vi "Autonomous Independent.vi"() -> ()   [LabVIEW 2012]
doc: "This VI is called when autonomous begins, and will automatically be terminated when autonomous ends. You can carry out timed or sensor driven robot movement independently without needing to return to the caller."
uses:
  <vilib>/Rock Robotics/WPI/Solenoid/WPI_SolenoidValue.ctl
  Robot Global Data.vi
  <vilib>/Rock Robotics/WPI/Solenoid/WPI_SolenoidSetEnum.vi
  <vilib>/Rock Robotics/WPI/Joystick/WPI_JoystickGetSetRefNum.vi
panel:
  in  "Shooter power 2":dbl=1.0
  in  "Shooter power":dbl=1.0
  in  "stop":bool
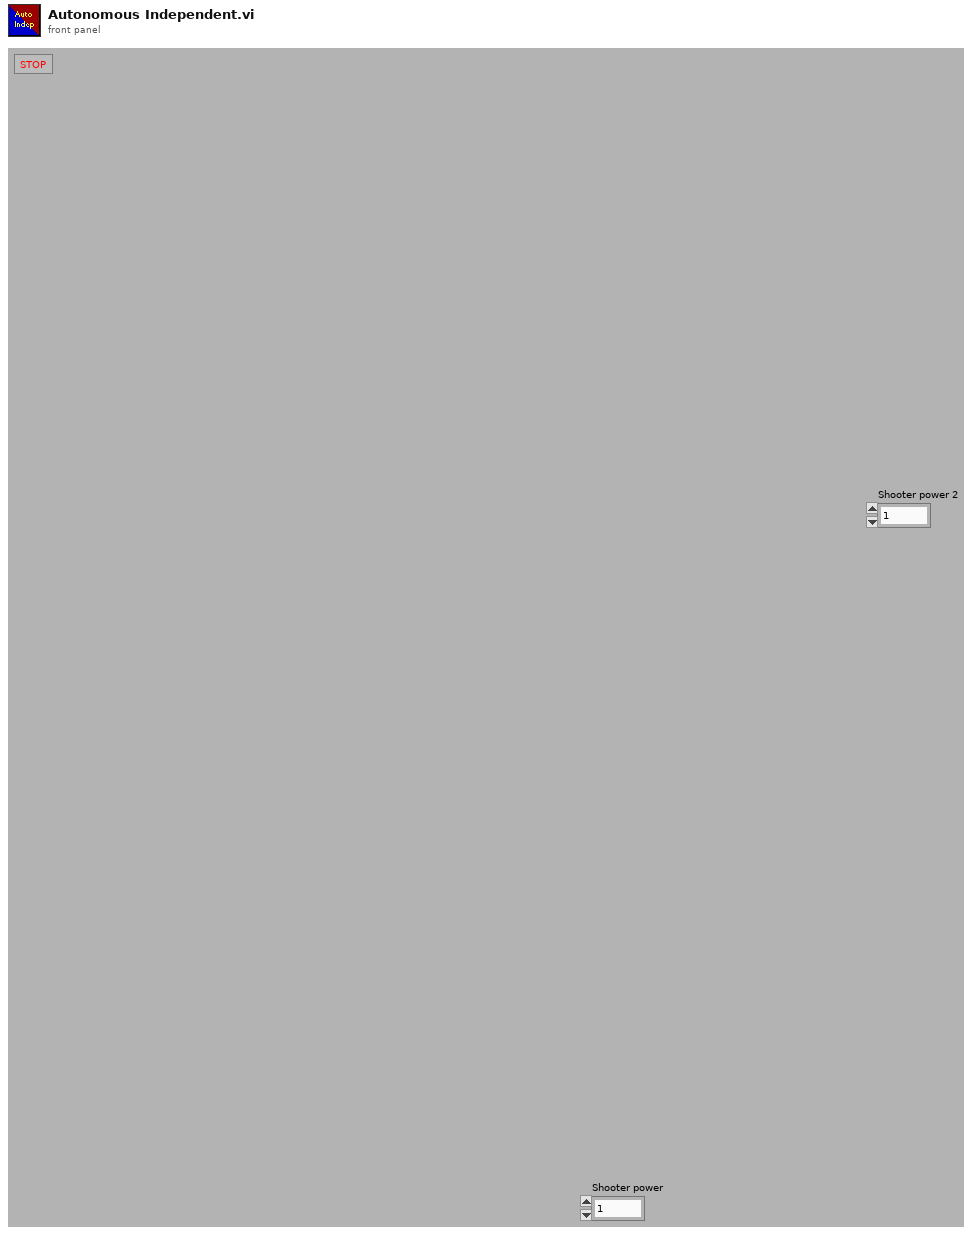
[diagram p1: front panel]
types:
  T1 = typedef "WPI_JoystickDevRef.ctl" = cluster{"Device":T2}
  T2 = typedef "WPI_JoystickDeviceEnum.ctl" = enum16{"USB 1", "USB 2", "USB 3", "USB 4", "Kinect 1", "Kinect 2"}
  T3 = cluster{"axis 1 (x)":dbl, "axis 2 (y)":dbl, "axis 3 (throttle)":dbl, "axis 4":dbl, "axis 5":dbl, "axis 6":dbl}
  T4 = typedef "WPI_SolenoidValue.ctl" = enum16{"Off", "On", "Forward", "Reverse"}
  T5 = typedef "WPI_MotorControlDeviceRef.ctl" = cluster{"DeviceStatus":errorcluster, "Type":enum16{"PWM", "CAN"}, "PWM":cluster{"Digital Module":T6, "PWM Channel":T7, "DeadBand":T8}, "CAN":cluster{"Device Number":u8, "Control Mode":T9, "Semaphore":T10, "Max Vout":dbl}, "Invert":bool, "TransformRef":T11, "InvTransformRef":T11}
  T6 = typedef "FPGA_TypedefDigitalModule.ctl" = enum16{"Digital Module 1", "Digital Module 2"}
  T7 = typedef "FPGA_DIOPWMChannel.ctl" = enum8{"PWM 1", "PWM 2", "PWM 3", "PWM 4", "PWM 5", "PWM 6", "PWM 7", "PWM 8", "PWM 9", "PWM 10", "Invalid"}
  T8 = typedef "WPI_PWMDeadband.ctl" = cluster{"Name":string, "maxPositivePwm":i32, "minPositivePwm":i32, "centerPwm":i32, "maxNegativePwm":i32, "minNegativePwm":i32, "angularRange":u16}
  T9 = typedef "WPI_CANJaguar_ControlMode.ctl" = enum8{"Percent VBus", "Current", "Speed", "Position", "Voltage"}
  T10 = typedef "Semaphore RefNum" = refnum<k1>
  T11 = typedef "WPI_PWMTransform_ConPane.ctl" = refnum<vi>
  T12 = typedef "WPI_SolenoidDevRef.ctl" = cluster{"DevStatus":errorcluster, "Solenoid Module":T13, "Forward Solenoid Channel":T14, "Reverse Solenoid Channel":T14}
  T13 = typedef "FPGA_TypedefSolenoidModule.ctl" = enum16{"Solenoid Module 1", "Solenoid Module 2"}
  T14 = typedef "WPI_SolenoidChannel.ctl" = enum8{"Solenoid 1", "Solenoid 2", "Solenoid 3", "Solenoid 4", "Solenoid 5", "Solenoid 6", "Solenoid 7", "Solenoid 8", "Invalid"}
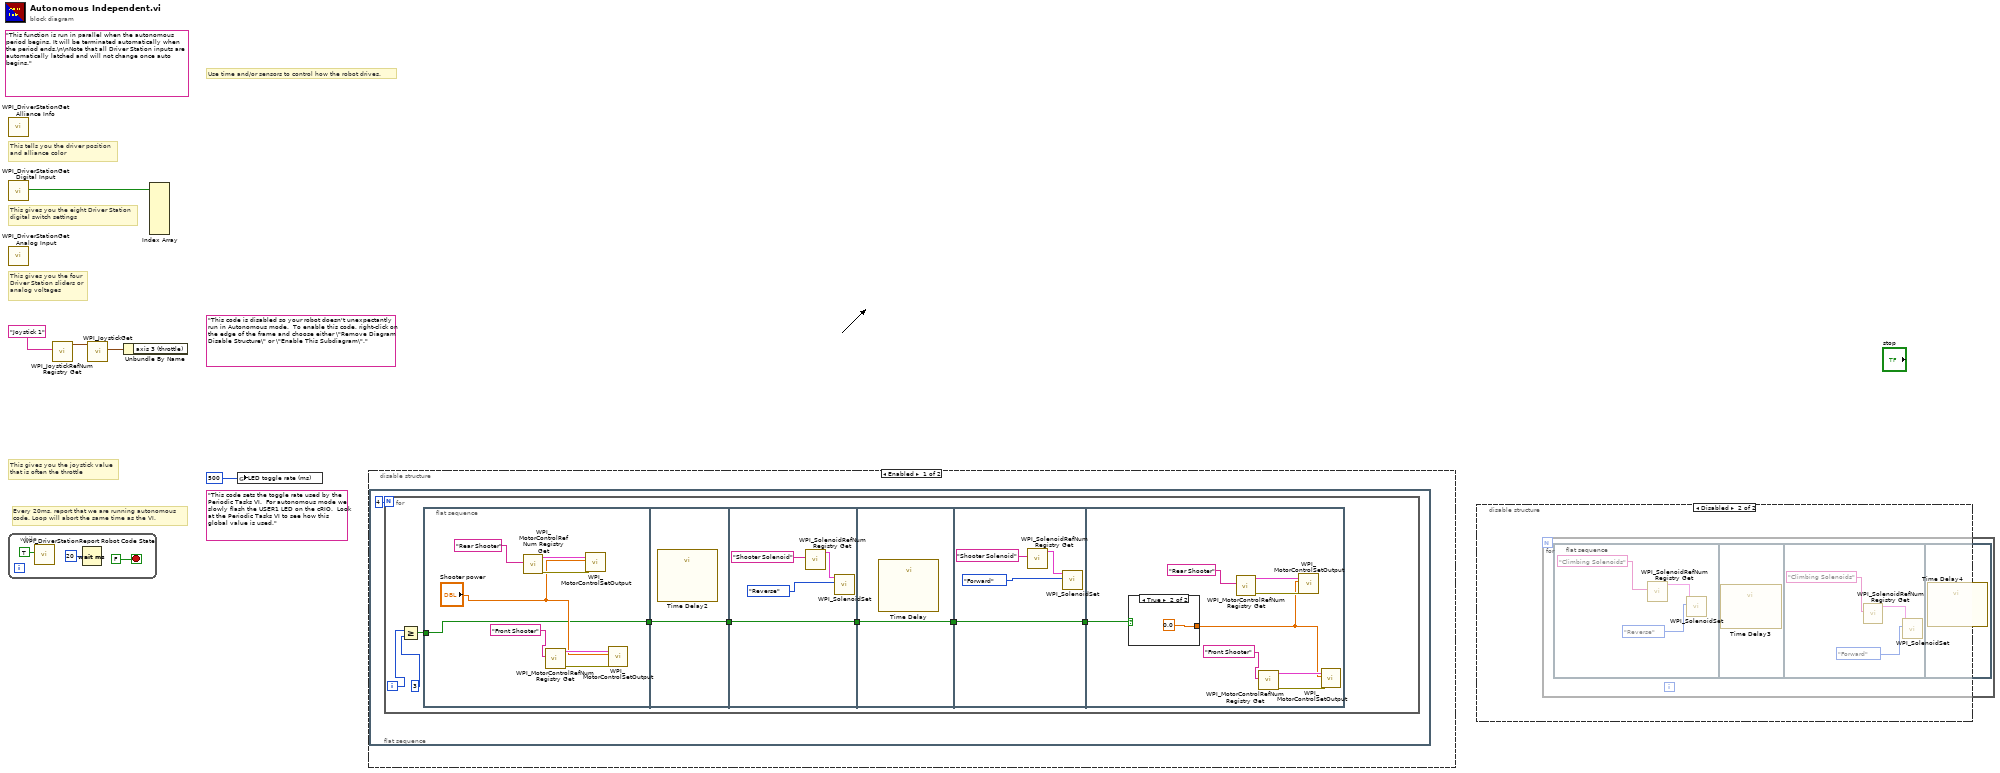
[diagram p0: block diagram]
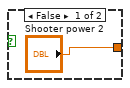
[diagram p3: hidden frame]
diagram:
  (unwired) "This code sets the toggle rate used by the Periodic Tasks VI.  For autonomous mode we slowly flash the USER1 LED on the cRIO.  Look at the Periodic Tasks VI to see how this global value is used."
  (unwired) "This code is disabled so your robot doesn't unexpectantly run in Autonomous mode.  To enable this code, right-click on the edge of the frame and choose either \"Remove Diagram Disable Structure\" or \"Enable This Subdiagram\"."
  (unwired) "This function is run in parallel when the autonomous period begins. It will be terminated automatically when the period ends.\n\nNote that all Driver Station inputs are automatically latched and will not change once auto begins."
  # "Every 20ms, report that we are running autonomous\ncode. Loop will abort the same time as the VI."
  # "This gives you the joystick value\nthat is often the throttle"
  # "Use time and/or sensors to control how the robot drives."
  # "This tells you the driver position\nand alliance color"
  # "This gives you the eight Driver Station\ndigital switch settings"
  # "This gives you the four\nDriver Station sliders or\nanalog voltages"
  n1 = while {
    stop <- FALSE stop-if-true
    n2 = call <vilib>:"WPI_DriverStationReport Robot Code State.vi"("Autonomous"=TRUE) -> ()  [unwired: 10 in, 1 out]
    n3 = Wait (ms)(milliseconds to wait=u32 20) -> ()  [unwired: 1 out]
  }
  n4 = call <vilib>:"WPI_DriverStationGet Alliance Info.vi"() -> ()  [unwired: 12 out]
  n5 = call <vilib>:"WPI_DriverStationGet Digital Input.vi"() -> ("Driver Station Digital Input (1-8)"=w5:bool[])  [unwired: 11 out]
  n6 = call <vilib>:"WPI_DriverStationGet Analog Input.vi"() -> ()  [unwired: 12 out]
  n7 = call <vilib>:"WPI_JoystickRefNum Registry Get.vi"("refnum name"="Joystick 1") -> ("JoystickDevRef"=w2:T1)  [unwired: 1 in, 9 out]
  n8 = call <vilib>:"WPI_JoystickGet.vi"("JoystickDevRef"=w2) -> ("Axes"=w3:T3)  [unwired: 1 in, 5 out]
  n9 = Unbundle By Name(w3) -> ()  [unwired: 1 out]
  n10 = Index Array(array=w5) -> ()  [unwired: 8 in, 8 out]
  n11 = global write "Robot Global Data.vi" "LED toggle rate (ms)"(u32 500 ("LED ms toggle rate")) -> ()
  n12 = disable-structure shown="Enabled" {
    frame Enabled {
      n13 = flat-sequence {
        frame #0 {
          n14 = for {
            N: 4 -> [_]
            i -> [w17]
            n15 = Greater Or Equal?(x=w17, y=3) -> (x >= y?=w10:bool)
            n16 = flat-sequence {
              tunnel: [w19] -> w16
              tunnel: w10 -> [w19]
              tunnel: w16 -> [w26]
              tunnel: [w26] -> w15
              tunnel: w15 -> [w27]
              tunnel: [w27] -> w14
              tunnel: w14 -> [w31]
              tunnel: [w31] -> w13
              tunnel: w13 -> [w32]
              tunnel: [w32] -> w12
              tunnel: w12 -> [w37]
              frame #0 {
                n17 = call <vilib>:"WPI_MotorControlRefNum Registry Get.vi"("refnum name"="Rear Shooter") -> ("error out"=w24:errorcluster, "MotorControlDevRef"=w25:T5)  [unwired: 9 in]
                n18 = call <vilib>:"WPI_MotorControlRefNum Registry Get.vi"("refnum name"="Front Shooter") -> ("error out"=w18:errorcluster, "MotorControlDevRef"=w23:T5)  [unwired: 9 in]
                n19 = call <vilib>:"WPI_MotorControlSetOutput.vi"("error in (no error)"=w24, "Output"="Shooter power", "MotorControlDevRef"=w25) -> ()  [unwired: 6 in, 3 out]
                n20 = call <vilib>:"WPI_MotorControlSetOutput.vi"("error in (no error)"=w18, "Output"="Shooter power", "MotorControlDevRef"=w23) -> ()  [unwired: 6 in, 3 out]
              }
              frame #1 {
                n21 = call "Time Delay2"() -> ()  [unwired: 11 in, 1 out]
              }
              frame #2 {
                n22 = call <vilib>:"WPI_SolenoidRefNum Registry Get.vi"("refnum name"="Shooter Solenoid") -> ("SolenoidDevRef"=w28:T12)  [unwired: 9 in, 1 out]
                n23 = call-poly <vilib>:"WPI_SolenoidSet.vi"("Value"=WPI_SolenoidValue."Reverse", "SolenoidDevRef"=w28) -> ()  [unwired: 8 in, 2 out]
              }
              frame #3 {
                n24 = call "Time Delay"() -> ()  [unwired: 11 in, 1 out]
              }
              frame #4 {
                n25 = call <vilib>:"WPI_SolenoidRefNum Registry Get.vi"("refnum name"="Shooter Solenoid") -> ("SolenoidDevRef"=w35:T12)  [unwired: 9 in, 1 out]
                n26 = call-poly <vilib>:"WPI_SolenoidSet.vi"("Value"=WPI_SolenoidValue."Forward", "SolenoidDevRef"=w35) -> ()  [unwired: 8 in, 2 out]
              }
              frame #5 {
                n27 = case shown="True" w37 {
                  tunnel: ["Shooter power 2" 0.0 ("Shooter power 2")] -> w38
                  frame False {
                  }
                  frame True {
                  }
                }
                n28 = call <vilib>:"WPI_MotorControlRefNum Registry Get.vi"("refnum name"="Rear Shooter") -> ("error out"=w42:errorcluster, "MotorControlDevRef"=w43:T5)  [unwired: 9 in]
                n29 = call <vilib>:"WPI_MotorControlRefNum Registry Get.vi"("refnum name"="Front Shooter") -> ("error out"=w40:errorcluster, "MotorControlDevRef"=w41:T5)  [unwired: 9 in]
                n30 = call <vilib>:"WPI_MotorControlSetOutput.vi"("error in (no error)"=w42, "Output"=w38, "MotorControlDevRef"=w43) -> ()  [unwired: 6 in, 3 out]
                n31 = call <vilib>:"WPI_MotorControlSetOutput.vi"("error in (no error)"=w40, "Output"=w38, "MotorControlDevRef"=w41) -> ()  [unwired: 6 in, 3 out]
              }
            }
          }
        }
      }
    }
    frame Disabled {
    }
  }
  n32 = disable-structure shown="Disabled" {
    frame Enabled {
    }
    frame Disabled {
      n33 = for {
        n34 = flat-sequence {
          frame #0 {
            n35 = call <vilib>:"WPI_SolenoidRefNum Registry Get.vi"("refnum name"="Climbing Solenoids") -> ("SolenoidDevRef"=w48:T12)  [unwired: 9 in, 1 out]
            n36 = call-poly <vilib>:"WPI_SolenoidSet.vi"("Value"=WPI_SolenoidValue."Reverse", "SolenoidDevRef"=w48) -> ()  [unwired: 8 in, 2 out]
          }
          frame #1 {
            n37 = call "Time Delay3"() -> ()  [unwired: 11 in, 1 out]
          }
          frame #2 {
            n38 = call <vilib>:"WPI_SolenoidRefNum Registry Get.vi"("refnum name"="Climbing Solenoids") -> ("SolenoidDevRef"=w51:T12)  [unwired: 9 in, 1 out]
            n39 = call-poly <vilib>:"WPI_SolenoidSet.vi"("Value"=WPI_SolenoidValue."Forward", "SolenoidDevRef"=w51) -> ()  [unwired: 8 in, 2 out]
          }
          frame #3 {
            n40 = call "Time Delay4"() -> ()  [unwired: 11 in, 1 out]
          }
        }
      }
    }
  }
